vi "FT10_FPGA_7854R_Main 2.vi"(5 "uSec Off":u16, 7 "uSec On":u16, 8 "Conn2/DIO_16_23 In":bool[](array[boolean])=[FALSE, FALSE, FALSE, FALSE, FALSE, FALSE, FALSE, FALSE], 9 "Conn2/DIO_8_15 In":bool[](array[boolean])=[FALSE, FALSE, FALSE, FALSE, FALSE, FALSE, FALSE, FALSE], 10 "Conn2/DIO_0_7 In":bool[](array[boolean])=[FALSE, FALSE, FALSE, FALSE, FALSE, FALSE, FALSE, FALSE], 11 "75kHz":bool) -> (0 "Conn2/DIO_16_23 Out":bool[](array[boolean]), 1 "Conn2/DIO_8_15 Out":bool[](array[boolean]), 2 "Conn2/DIO_0_7 Out":bool[](array[boolean]))   [LabVIEW 2024]
uses:
  <vilib>/rvi/Emulation/niFpgaGetClockAttributes.vi
  <vilib>/rvi/Emulation/niFpgaSctlEmulationGetInTimedLoop.vi
  <vilib>/rvi/Emulation/niFpgaEmulationReportErrorSimple.vi
  <vilib>/rvi/eio/common/nirviEmuTemplateMethod_errors.vi
  <vilib>/rvi/Emulation/niFpgaCriticalErrorInLSC.vi
  <vilib>/eio/EIONode/EIONode.xnode
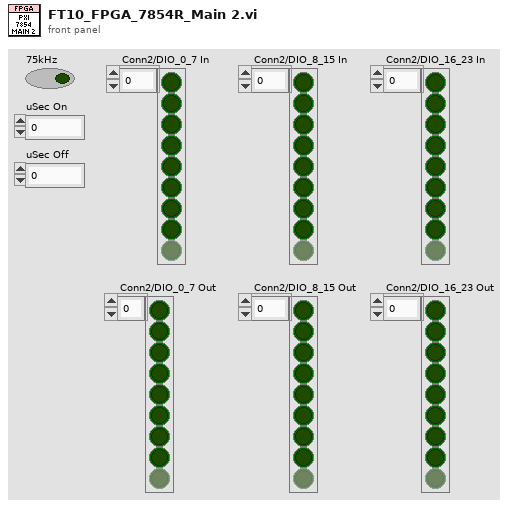
[diagram p1: front panel]
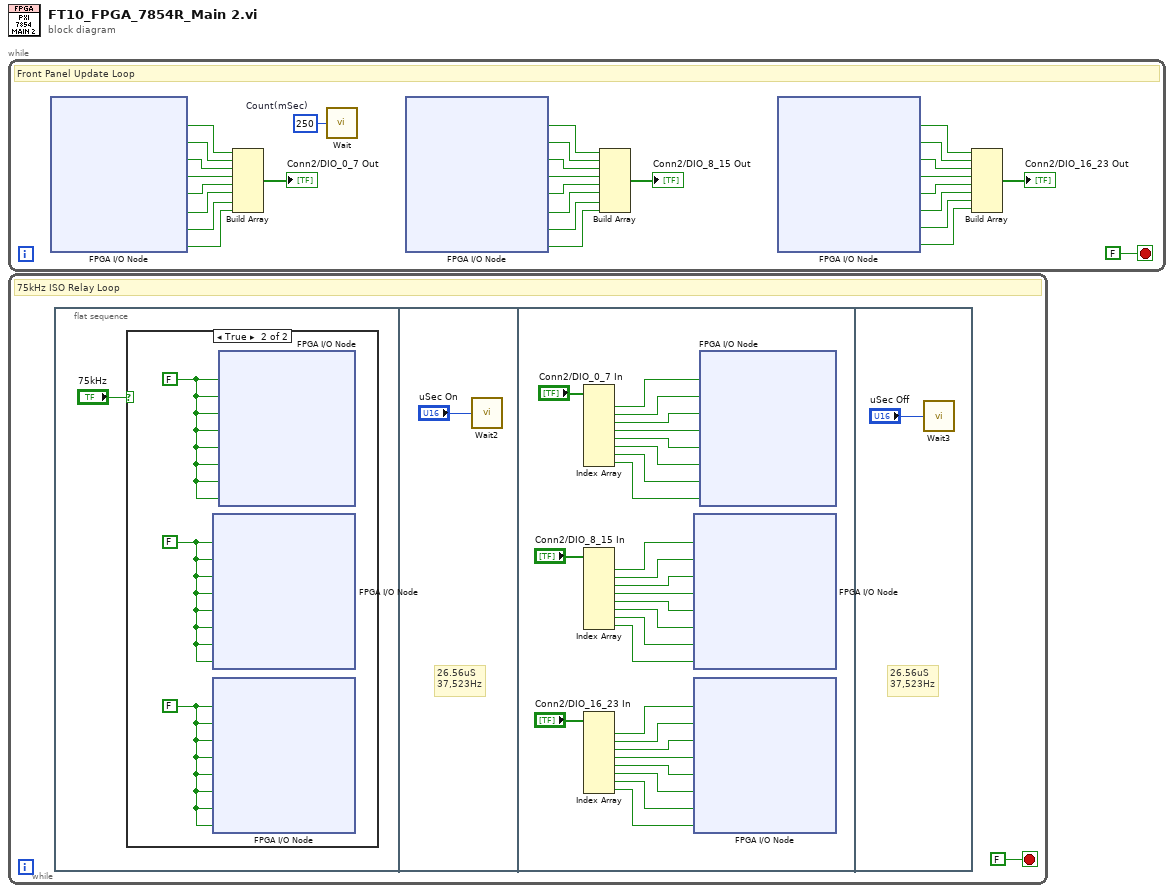
[diagram p0: block diagram]
diagram:
  n1 = while {
    stop <- FALSE stop-if-true
    w28 = u8 250  # Count(mSec)
    # "Front Panel Update Loop"
    n2 = xnode "FPGA I/O Node"() -> ("Connector2/DIO0"=w27:bool, "Connector2/DIO1"=w26:bool, "Connector2/DIO2"=w25:bool, "Connector2/DIO3"=w24:bool, "Connector2/DIO4"=w23:bool, "Connector2/DIO5"=w22:bool, "Connector2/DIO6"=w21:bool, "Connector2/DIO7"=w20:bool)  [unwired: 8 in, 8 out]
    n3 = Build Array(w27, w26, w25, w24, w23, w22, w21, w20) -> (→"Conn2/DIO_0_7 Out":bool[])
    n4 = call "Wait"("Count(mSec)"=w28) -> ()  [unwired: 1 out]
    n5 = xnode "FPGA I/O Node"() -> ("Connector2/DIO8"=w18:bool, "Connector2/DIO9"=w17:bool, "Connector2/DIO10"=w16:bool, "Connector2/DIO11"=w15:bool, "Connector2/DIO12"=w14:bool, "Connector2/DIO13"=w13:bool, "Connector2/DIO14"=w12:bool, "Connector2/DIO15"=w11:bool)  [unwired: 8 in, 8 out]
    n6 = Build Array(w18, w17, w16, w15, w14, w13, w12, w11) -> (→"Conn2/DIO_8_15 Out":bool[])
    n7 = xnode "FPGA I/O Node"() -> ("Connector2/DIO16"=w9:bool, "Connector2/DIO17"=w7:bool, "Connector2/DIO18"=w6:bool, "Connector2/DIO19"=w5:bool, "Connector2/DIO20"=w1:bool, "Connector2/DIO21"=w2:bool, "Connector2/DIO22"=w3:bool, "Connector2/DIO23"=w4:bool)  [unwired: 8 in, 8 out]
    n8 = Build Array(w9, w7, w6, w5, w1, w2, w3, w4) -> (→"Conn2/DIO_16_23 Out":bool[])
  }
  n9 = while {
    stop <- FALSE stop-if-true
    # "75kHz ISO Relay Loop"
    n10 = flat-sequence {
      frame #0 {
        n11 = case shown="True" "75kHz" {
          frame False {
          }
          frame True {
            w32 = FALSE ("Connector2/DIO8")
            w34 = FALSE ("Connector2/DIO8")
            w33 = FALSE ("Connector2/DIO0")
            n12 = xnode "FPGA I/O Node"("Connector2/DIO8"=w34, "Connector2/DIO9"=w34, "Connector2/DIO10"=w34, "Connector2/DIO11"=w34, "Connector2/DIO12"=w34, "Connector2/DIO13"=w34, "Connector2/DIO14"=w34, "Connector2/DIO15"=w34) -> ()  [unwired: 8 in, 8 out]
            n13 = xnode "FPGA I/O Node"("Connector2/DIO16"=w32, "Connector2/DIO17"=w32, "Connector2/DIO18"=w32, "Connector2/DIO19"=w32, "Connector2/DIO20"=w32, "Connector2/DIO21"=w32, "Connector2/DIO22"=w32, "Connector2/DIO23"=w32) -> ()  [unwired: 8 in, 8 out]
            n14 = xnode "FPGA I/O Node"("Connector2/DIO0"=w33, "Connector2/DIO1"=w33, "Connector2/DIO2"=w33, "Connector2/DIO3"=w33, "Connector2/DIO4"=w33, "Connector2/DIO5"=w33, "Connector2/DIO6"=w33, "Connector2/DIO7"=w33) -> ()  [unwired: 8 in, 8 out]
          }
        }
      }
      frame #1 {
        # "26.56uS\n37,523Hz"
        n15 = call "Wait2"("Count(uSec)"="uSec On") -> ()  [unwired: 1 out]
      }
      frame #2 {
        n16 = Index Array(array="Conn2/DIO_0_7 In") -> (element #1=w60:bool, element #2=w59:bool, element #3=w58:bool, element #4=w57:bool, element #5=w56:bool, element #6=w55:bool, element #7=w54:bool, element #8=w53:bool)  [unwired: 8 in]
        n17 = Index Array(array="Conn2/DIO_8_15 In") -> (element #1=w52:bool, element #2=w51:bool, element #3=w50:bool, element #4=w49:bool, element #5=w48:bool, element #6=w47:bool, element #7=w46:bool, element #8=w45:bool)  [unwired: 8 in]
        n18 = Index Array(array="Conn2/DIO_16_23 In") -> (element #1=w43:bool, element #2=w42:bool, element #3=w41:bool, element #4=w40:bool, element #5=w39:bool, element #6=w38:bool, element #7=w37:bool, element #8=w36:bool)  [unwired: 8 in]
        n19 = xnode "FPGA I/O Node"("Connector2/DIO8"=w52, "Connector2/DIO9"=w51, "Connector2/DIO10"=w50, "Connector2/DIO11"=w49, "Connector2/DIO12"=w48, "Connector2/DIO13"=w47, "Connector2/DIO14"=w46, "Connector2/DIO15"=w45) -> ()  [unwired: 8 in, 8 out]
        n20 = xnode "FPGA I/O Node"("Connector2/DIO16"=w43, "Connector2/DIO17"=w42, "Connector2/DIO18"=w41, "Connector2/DIO19"=w40, "Connector2/DIO20"=w39, "Connector2/DIO21"=w38, "Connector2/DIO22"=w37, "Connector2/DIO23"=w36) -> ()  [unwired: 8 in, 8 out]
        n21 = xnode "FPGA I/O Node"("Connector2/DIO0"=w60, "Connector2/DIO1"=w59, "Connector2/DIO2"=w58, "Connector2/DIO3"=w57, "Connector2/DIO4"=w56, "Connector2/DIO5"=w55, "Connector2/DIO6"=w54, "Connector2/DIO7"=w53) -> ()  [unwired: 8 in, 8 out]
      }
      frame #3 {
        # "26.56uS\n37,523Hz"
        n22 = call "Wait3"("Count(uSec)"="uSec Off") -> ()  [unwired: 1 out]
      }
    }
  }
